vi "waveform player.vi"(1 "notifier name":string="wave out") -> ()   [LabVIEW 2009]
uses:
  event notifier.ctl
  <vilib>/sound/lvsound.llb/Sound Format.ctl
panel:
  out "type":T1(ring)
  out "buffer writes":i32
  out "notifier iterations":i32
  in  "STOP":bool
  in  "mono 8-bit":u8[](array[slide]) scale=0.0..255.0
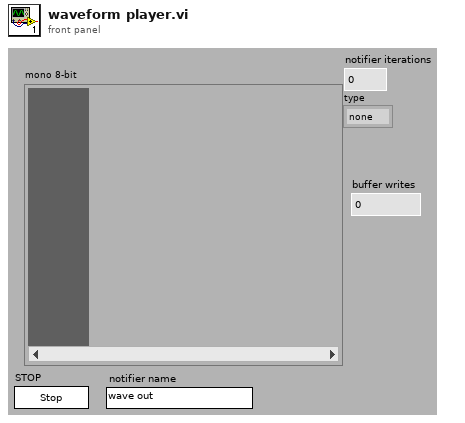
[diagram p1: front panel]
types:
  T1 = enum8{"none", "end", "start", "pause", "update", "volume"}
  T2 = typedef "event notifier.ctl" = cluster{"type":enum8{"none", "end", "start", "pause", "update", "volume"}, "message":string}
  T3 = typedef "Sound Format.ctl" = cluster{"sound quality":enum16{"mono", "stereo"}, "rate":enum16{"11025", "22050", "44100", "8000"}, "bits per sample":enum16{"8 bit", "16 bit"}}
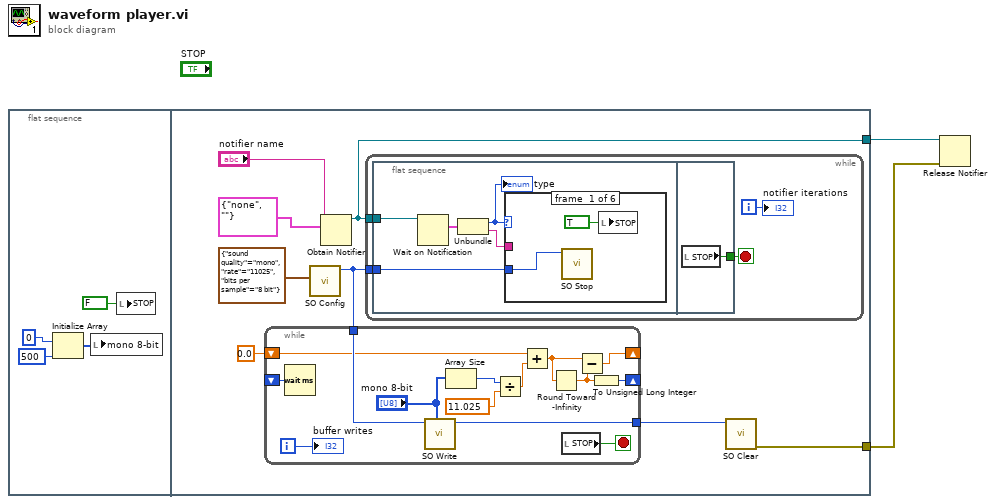
[diagram p0: block diagram]
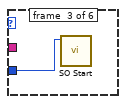
[diagram p3: hidden frame]
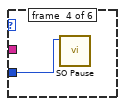
[diagram p4: hidden frame]
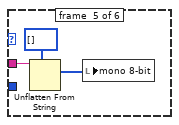
[diagram p5: hidden frame]
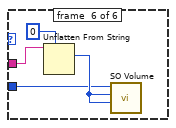
[diagram p6: hidden frame]
diagram:
  n1 = flat-sequence {
    tunnel: [w8] -> w2
    tunnel: [w7] -> w1
    frame #0 {
      n2 = Initialize Array(u8 0, 500) -> (w5:u8[])
      n3 = local write "mono 8-bit"(w5) -> ()
      n4 = local write "STOP"(FALSE ("STOP")) -> ()
    }
    frame #1 {
      n5 = call <vilib>:"SO Config.vi"("sound format"=T3 {"sound quality"=enum."mono", "rate"=enum."11025", "bits per sample"=enum."8 bit"}) -> ("task ID out"=w9:u32)  [unwired: 9 in, 1 out]
      n6 = while {
        tunnel: w9 -> [w49]
        tunnel: [w47] -> w13
        shift-right: [w41] -> _
        shift-left: 0.0 -> [w43]
        shift-right: [w39] -> _
        shift-left: _ -> [w38]
        i -> [w36]
        stop <- w37 stop-if-true
        n7 = Wait (ms)(milliseconds to wait=w38) -> ()  [unwired: 1 out]
        n8 = call <vilib>:"SO Write.vi"("mono 8-bit"="mono 8-bit", "task ID in"=w49) -> ("task ID out"=w47:u32)  [unwired: 8 in, 1 out]
        n9 = Array Size(array="mono 8-bit") -> (size(s)=w45:i32)
        n10 = Divide(x=w45, y=11.025) -> (x/y=w44:dbl)
        n11 = Add(x=w43, y=w44) -> (x+y=w42:dbl)
        n12 = Round Toward -Infinity(1:w42) -> (0:w40:dbl)
        n13 = local read "STOP"() -> (w37:bool)
        n14 = Subtract(x=w42, y=w40) -> (x-y=w41:dbl)
        n15 = To Unsigned Long Integer(number=w40) -> (unsigned 32bit integer=w39:u32)
        "buffer writes" <- w36
      }
      n16 = Obtain Notifier(name (unnamed)="notifier name", notification data type=T2 {"type"=enum."none", "message"=""} ("notification")) -> (notifier out=w8:refnum<notifier>)  [unwired: 2 in, 2 out]
      n17 = while {
        tunnel: w9 -> [w17]
        tunnel: w8 -> [w18]
        i -> [w15]
        stop <- w16 stop-if-true
        n18 = flat-sequence {
          tunnel: w18 -> [w23]
          tunnel: w17 -> [w21]
          tunnel: [w35] -> w16
          frame #0 {
            n19 = Wait on Notification(notifier=w23) -> (notification=w22:T2)  [unwired: 3 in, 3 out]
            n20 = Unbundle(w22) -> ("type"=w19:T1, "message"=w20:string)
            "type" <- w19
            n21 = case shown="\"start\"" w19 {
              tunnel: w21 -> [w24 _ w26 w27 _ w31]
              tunnel: w20 -> [_ _ _ _ w30 w34]
              frame #0 {
                n22 = call <vilib>:"SO Stop.vi"("task ID in"=w24) -> ()  [unwired: 9 in, 2 out]
                n23 = local write "STOP"(TRUE ("STOP")) -> ()
              }
              frame #1 {
              }
              frame #2 {
                n24 = call <vilib>:"SO Start.vi"("task ID in"=w26) -> ()  [unwired: 9 in, 2 out]
              }
              frame #3 {
                n25 = call <vilib>:"SO Pause.vi"("task ID in"=w27) -> ()  [unwired: 9 in, 2 out]
              }
              frame #4 {
                n26 = Unflatten From String(type=u8[] [] ("mono 8-bit"), binary string=w30) -> (value=w28:u8[])  [unwired: 3 in, 2 out]
                n27 = local write "mono 8-bit"(w28) -> ()
              }
              frame #5 {
                n28 = Unflatten From String(type=u16 0 ("left channel"), binary string=w34) -> (value=w32:u16)  [unwired: 3 in, 2 out]
                n29 = call <vilib>:"SO Volume.vi"("right channel"=w32, "left channel"=w32, "task ID in"=w31) -> ()  [unwired: 7 in, 2 out]
              }
            }
          }
          frame #1 {
            n30 = local read "STOP"() -> (w35:bool)
          }
        }
        "notifier iterations" <- w15
      }
      n31 = call <vilib>:"SO Clear.vi"("task ID in"=w13) -> ("error out"=w7:errorcluster)  [unwired: 10 in]
    }
  }
  n32 = Release Notifier(notifier=w2, error in (no error)=w1) -> ()  [unwired: 1 in, 3 out]
